vi "HEWH Analyze Total.vi"(7 "Test Type":T6, 8 "error in (no error)":errorcluster, 11 "UEF Calculated Values Input":T1 {"Data Indexes"."15 sec after Draw Index" format="%#.2f"; "Data Indexes"."15 sec after Draw Timestamp" format="%#.2f"; "Data Indexes"."Test Start Timestamp" format="%.2f"; "Data Indexes"."Test End Timestamp" format="%.2f"; "Data Indexes"."T0 Timestamp" format="%.2f"; "Data Indexes"."Tsf Timestamp" format="%.2f"; "Data Indexes"."Tsu0 Timestamp" format="%.2f"; "Data Indexes"."Tmax1 Timestamp" format="%.2f"; "Data Indexes"."Draw Index Timestamp" format="%#.2f"; "Data Indexes"."Non-Draw Timestamp" format="%#.2f"; "Data Indexes"."Heating Timestamp" format="%#.2f"; "Data Indexes"."Start Energy (BTU-Gas)" format="%.6f"; "Data Indexes"."Start Watt Hours" format="%.6f"; "Static Data"."V - Volume of Wh (True)" format="%.5f"; "Static Data"."T-Ambinet Nominal (°F)" format="%.5f"; "Static Data"."T-Inlet Setpoint (°F)" format="%.5f"; "Static Data"."T-Wh Setpoint (°F)" format="%.5f"; "Sampled Data"."Qe (Wh)" format="%.5f"; "Sampled Data"."Tau stby2 (hr)" format="%.5f"; "Sampled Data"."Tastby2 (°F)" format="%.5f"; "Sampled Data"."Qf (BTU)" format="%.5f"; "Sampled Data"."Qe (BTU)" format="%.5f"; "Sampled Data"."Tmax1 (°F)" format="%.5f"; "Sampled Data"."T0 (°F)" format="%.5f"; "Sampled Data"."Qr (BTU)" format="%.5f"; "Sampled Data"."T 24(°F)" format="%.5f"; "Sampled Data"."T astby(°F)" format="%.5f"; "Sampled Data"."T tstby(°F)" format="%.5f"; "Sampled Data"."T su0(°F)" format="%.5f"; "Sampled Data"."T suf(°F)" format="%.5f"; "Sampled Data"."Tau stby_1 (hr)" format="%.5f"; "Sampled Data"."Qsuf (BTU)" format="%.5f"; "Sampled Data"."Qsu0 (BTU)" format="%.5f"; "Calculated Values"."Draw Bonus Volume (gal)" format="%.6f"; "Calculated Values"."Adjustment Factor" format="%.6f"; "Calculated Values"."T*avg_del(n-1)" format="%.6f"; "Calculated Values"."T*min(n-1)" format="%.6f"; "Calculated Values"."T*avg_del(n)" format="%.6f"; "Calculated Values"."Vn" format="%.6f"; "Calculated Values"."Qdm (BTU)" format="%.6f"; "Calculated Values"."QHWD (BTU)" format="%.6f"; "Calculated Values"."QHW (BTU)" format="%.6f"; "Calculated Values"."UEF" format="%.6f"; "Calculated Values"."QHW67 (BTU)" format="%.6f"; "Calculated Values"."Qda (BTU)" format="%.6f"; "Calculated Values"."Qd (BTU)" format="%.6f"; "Calculated Values"."Q (BTU)" format="%.6f"; "Calculated Values"."UA (BTU/(hr*F))" format="%.6f"; "Calculated Values"."Qhr (BTU/hr)" format="%.6f"; "Calculated Values"."Qstby (BTU)" format="%.6f"; "Calculated Values"."nu_r" format="%.6f"; "Calculated Values"."CpUEF (BTU/(lb*F))" format="%.6f"; "Calculated Values"."rho_nu (lb/gal)" format="%.6f"; "Calculated Values"."V1- Vol (Gal)" format="%.6f"; "Calculated Values"."M cluster mass removed (lb)" format="%.6f"; "Calculated Values"."Cp theoretical (BTU/(lbm °F))" format="%.6f"; "Calculated Values"."Tin1 - Mean Inlet 1st Cluster (°F)" format="%.6f"; "Calculated Values"."Tdel1-Mean Outlet 1st Cluster(°F)" format="%.6f"; "Calculated Values"."Cp 24 (BTU/(lb*F))" format="%.6f"; "Calculated Values"."Cp standby (BTU/(lb*F))" format="%.6f"; "Calculated Values"."Cp2 (BTU/(lb*F))" format="%.6f"; "Calculated Values"."Cp1 (BTU/(lb*F))" format="%.6f"; "Calculated Values"."rho 24 (lb/gal)" format="%.6f"; "Calculated Values"."rho standby (lb/gal)" format="%.6f"; "Calculated Values"."rho 2 (lb/gal)" format="%.6f"; "Calculated Values"."Density of cold water All (lbm/gal)" format="%#.3g"; "Calculated Values"."CpHW (BTU/(lbm °F))" format="%#.3g"; "Calculated Values"."Density of hot water All (lbm/gal)" format="%#.3g"; "Calculated Values"."Mass of water All (lbm)" format="%#.3f"}) -> (0 "error out":errorcluster, 3 "UEF Calculated Values Output":T1 {"Data Indexes"."15 sec after Draw Index" format="%#.2f"; "Data Indexes"."15 sec after Draw Timestamp" format="%#.2f"; "Data Indexes"."Test Start Timestamp" format="%.2f"; "Data Indexes"."Test End Timestamp" format="%.2f"; "Data Indexes"."T0 Timestamp" format="%.2f"; "Data Indexes"."Tsf Timestamp" format="%.2f"; "Data Indexes"."Tsu0 Timestamp" format="%.2f"; "Data Indexes"."Tmax1 Timestamp" format="%.2f"; "Data Indexes"."Draw Index Timestamp" format="%#.2f"; "Data Indexes"."Non-Draw Timestamp" format="%#.2f"; "Data Indexes"."Heating Timestamp" format="%#.2f"; "Data Indexes"."Start Energy (BTU-Gas)" format="%.6f"; "Data Indexes"."Start Watt Hours" format="%.6f"; "Static Data"."V - Volume of Wh (True)" format="%.5f"; "Static Data"."T-Ambinet Nominal (°F)" format="%.5f"; "Static Data"."T-Inlet Setpoint (°F)" format="%.5f"; "Static Data"."T-Wh Setpoint (°F)" format="%.5f"; "Sampled Data"."Qe (Wh)" format="%.5f"; "Sampled Data"."Tau stby2 (hr)" format="%.5f"; "Sampled Data"."Tastby2 (°F)" format="%.5f"; "Sampled Data"."Qf (BTU)" format="%.5f"; "Sampled Data"."Qe (BTU)" format="%.5f"; "Sampled Data"."Tmax1 (°F)" format="%.5f"; "Sampled Data"."T0 (°F)" format="%.5f"; "Sampled Data"."Qr (BTU)" format="%.5f"; "Sampled Data"."T 24(°F)" format="%.5f"; "Sampled Data"."T astby(°F)" format="%.5f"; "Sampled Data"."T tstby(°F)" format="%.5f"; "Sampled Data"."T su0(°F)" format="%.5f"; "Sampled Data"."T suf(°F)" format="%.5f"; "Sampled Data"."Tau stby_1 (hr)" format="%.5f"; "Sampled Data"."Qsuf (BTU)" format="%.5f"; "Sampled Data"."Qsu0 (BTU)" format="%.5f"; "Calculated Values"."Draw Bonus Volume (gal)" format="%.6f"; "Calculated Values"."Adjustment Factor" format="%.6f"; "Calculated Values"."T*avg_del(n-1)" format="%.6f"; "Calculated Values"."T*min(n-1)" format="%.6f"; "Calculated Values"."T*avg_del(n)" format="%.6f"; "Calculated Values"."Vn" format="%.6f"; "Calculated Values"."Qdm (BTU)" format="%.6f"; "Calculated Values"."QHWD (BTU)" format="%.6f"; "Calculated Values"."QHW (BTU)" format="%.6f"; "Calculated Values"."UEF" format="%.6f"; "Calculated Values"."QHW67 (BTU)" format="%.6f"; "Calculated Values"."Qda (BTU)" format="%.6f"; "Calculated Values"."Qd (BTU)" format="%.6f"; "Calculated Values"."Q (BTU)" format="%.6f"; "Calculated Values"."UA (BTU/(hr*F))" format="%.6f"; "Calculated Values"."Qhr (BTU/hr)" format="%.6f"; "Calculated Values"."Qstby (BTU)" format="%.6f"; "Calculated Values"."nu_r" format="%.6f"; "Calculated Values"."CpUEF (BTU/(lb*F))" format="%.6f"; "Calculated Values"."rho_nu (lb/gal)" format="%.6f"; "Calculated Values"."V1- Vol (Gal)" format="%.6f"; "Calculated Values"."M cluster mass removed (lb)" format="%.6f"; "Calculated Values"."Cp theoretical (BTU/(lbm °F))" format="%.6f"; "Calculated Values"."Tin1 - Mean Inlet 1st Cluster (°F)" format="%.6f"; "Calculated Values"."Tdel1-Mean Outlet 1st Cluster(°F)" format="%.6f"; "Calculated Values"."Cp 24 (BTU/(lb*F))" format="%.6f"; "Calculated Values"."Cp standby (BTU/(lb*F))" format="%.6f"; "Calculated Values"."Cp2 (BTU/(lb*F))" format="%.6f"; "Calculated Values"."Cp1 (BTU/(lb*F))" format="%.6f"; "Calculated Values"."rho 24 (lb/gal)" format="%.6f"; "Calculated Values"."rho standby (lb/gal)" format="%.6f"; "Calculated Values"."rho 2 (lb/gal)" format="%.6f"; "Calculated Values"."Density of cold water All (lbm/gal)" format="%#.3g"; "Calculated Values"."CpHW (BTU/(lbm °F))" format="%#.3g"; "Calculated Values"."Density of hot water All (lbm/gal)" format="%#.3g"; "Calculated Values"."Mass of water All (lbm)" format="%#.3f"})   [LabVIEW 2023]
uses:
  Type Definitions/UEF Constants.ctl
  Type Definitions/HEWH Draw Stats.ctl
  Type Definitions/HEWH FHR Draw Type.ctl
  Type Definitions/FHR Bins.ctl
  Type Definitions/HEWH Meter Type.ctl
  Type Definitions/HEWH Test Type.ctl
  <vilib>/Utility/error.llb/whitespace.ctl
  <vilib>/Utility/error.llb/Trim Whitespace One-Sided.vi
panel:
  out "Sampled Data.Hot Water Draw Amounts-(Gal)":dbl[](array[numeric])
  out "output variable":dbl
  # "FHR"
  # "FHR"
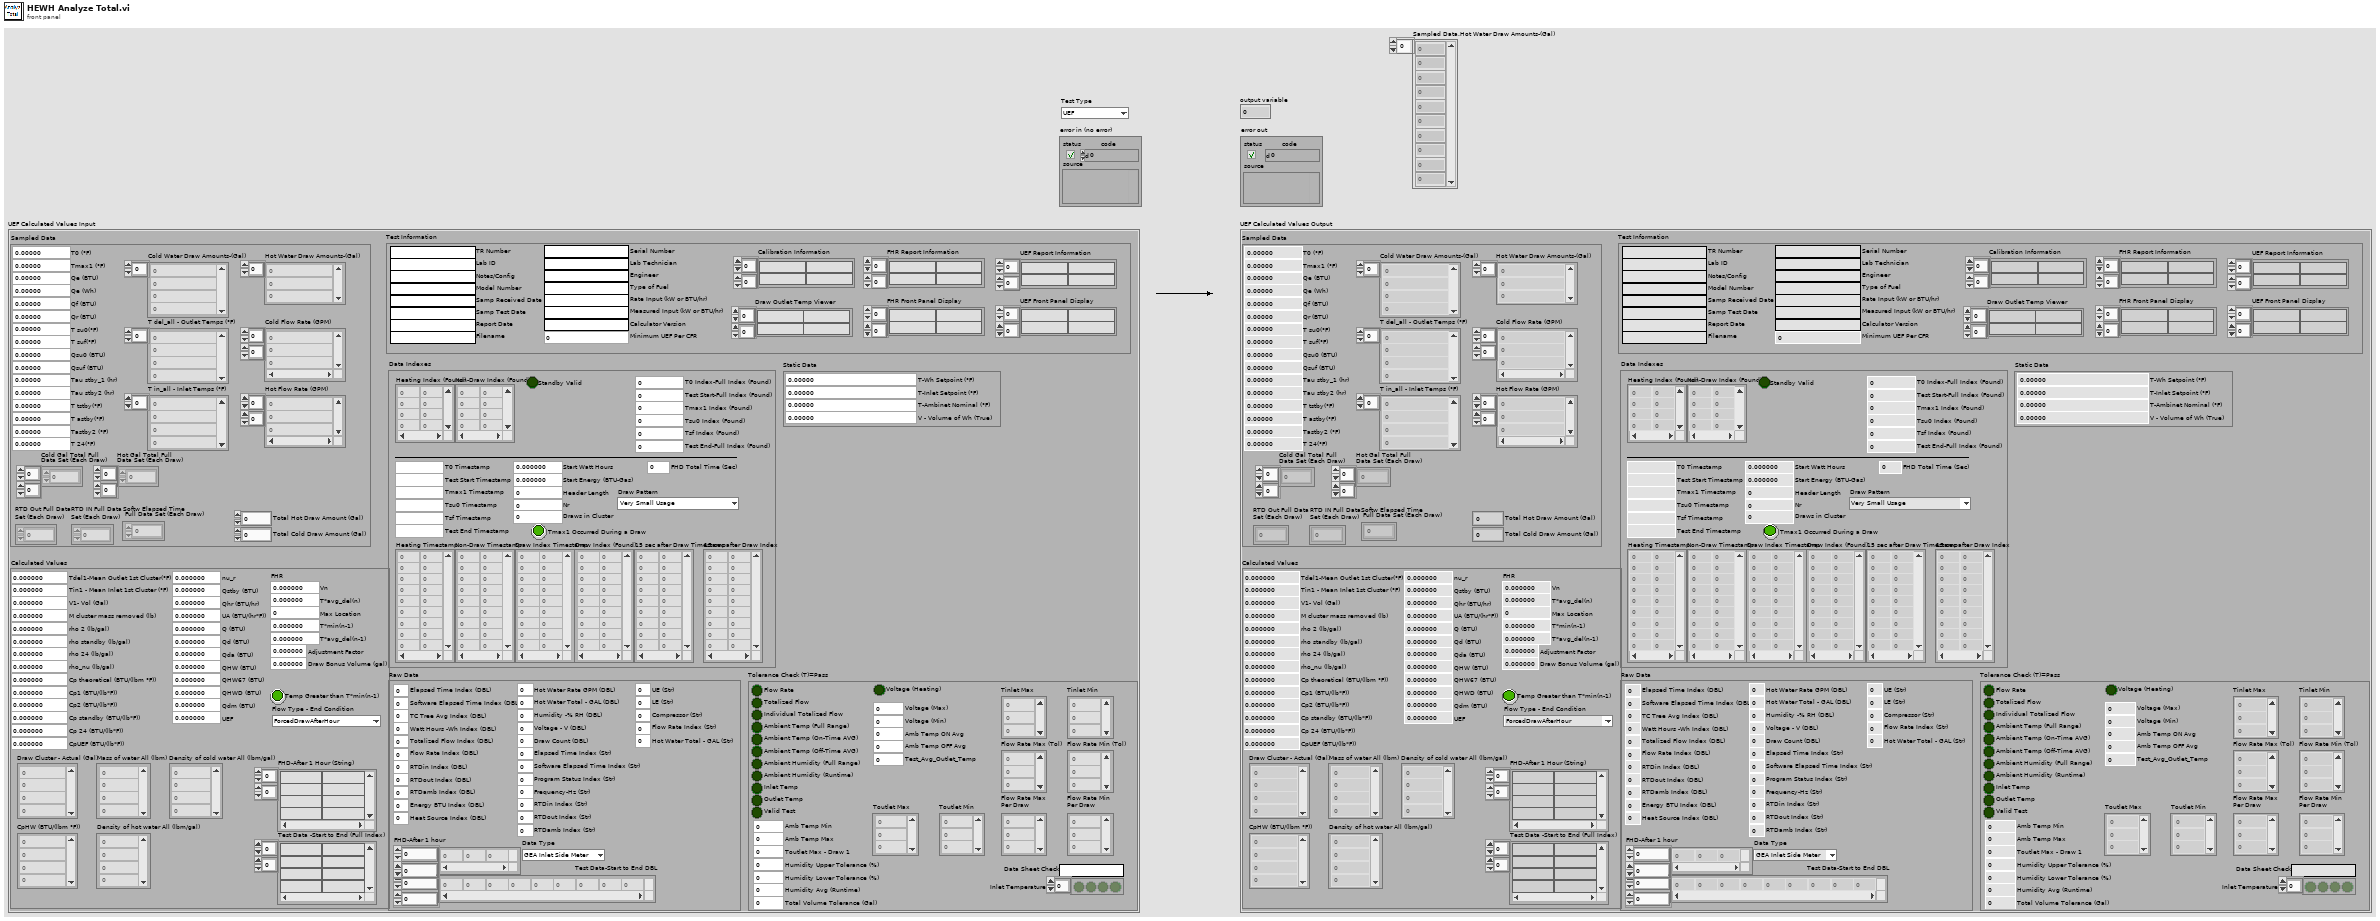
[diagram p1: front panel]
types:
  T1 = typedef "UEF Constants.ctl" = cluster{"Calculated Values":T2, "Sampled Data":cluster{"Cold Water Draw Amounts-(Gal)":dbl[], "T del_all - Outlet Temps (°F)":dbl[], "T in_all - Inlet Temps (°F)":dbl[], "Qsu0 (BTU)":dbl, "Qsuf (BTU)":dbl, "Tau stby_1 (hr)":dbl, "T suf(°F)":dbl, "T su0(°F)":dbl, "T tstby(°F)":dbl, "T astby(°F)":dbl, "T 24(°F)":dbl, "Qr (BTU)":dbl, "T0 (°F)":dbl, "Tmax1 (°F)":dbl, "Qe (BTU)":dbl, "Qf (BTU)":dbl, "Tastby2 (°F)":dbl, "RTD Out Full Data\nSet (Each Draw)":dbl[][], "RTD IN Full Data\nSet (Each Draw)":dbl[][], "Tau stby2 (hr)":dbl, "Hot Water Draw Amounts-(Gal)":dbl[], "Cold Flow Rate (GPM)":dbl[][], "Hot Flow Rate (GPM)":dbl[][], "Softw Elapsed Time\n Full Data Set (Each Draw)":dbl[][], "Cold Gal Total Full\nData Set (Each Draw)":dbl[][], "Total Hot Draw Amount (Gal) ":dbl, "Total Cold Draw Amount (Gal)":dbl, "Qe (Wh)":dbl, "Hot Gal Total Full\nData Set (Each Draw)":dbl[][]}, "Static Data":cluster{"T-Wh Setpoint (°F)":dbl, "T-Inlet Setpoint (°F)":dbl, "T-Ambinet Nominal (°F)":dbl, "V - Volume of Wh (True)":dbl}, "Data Indexes":cluster{"Test Start-Full Index (Found)":i32, "Header Length":i32, "Draw Index (Found)":i32[][], "Nr":i32, "Start Watt Hours":dbl, "Tsu0 Index (Found)":i32, "Tsf Index (Found)":i32, "Start Energy (BTU-Gas)":dbl, "Draws in Cluster":i32, "T0 Index-Full Index (Found)":i32, "Non-Draw Index (Found)":i32[][], "Tmax1 Index (Found)":i32, "Test End-Full Index (Found)":i32, "Heating Index (Found)":i32[][], "Heating Timestamp":dbl[][], "Non-Draw Timestamp":dbl[][], "Draw Index Timestamp":dbl[][], "Tmax1 Timestamp":dbl, "Tsu0 Timestamp":dbl, "Tsf Timestamp":dbl, "T0 Timestamp":dbl, "Test End Timestamp":dbl, "Test Start Timestamp":dbl, "15 sec after Draw Timestamp":dbl[][], "15 sec after Draw Index":dbl[][], "Tmax1 Occurred During a Draw":bool, "FHD Total Time (Sec)":dbl, "Draw Pattern":T4, "Standby Valid":bool}, "Raw Data":cluster{"Elapsed Time Index (DBL)":i32, "Software Elapsed Time Index (DBL)":i32, "TC Tree Avg Index (DBL)":i32, "Watt Hours -Wh Index (DBL)":i32, "Energy BTU Index (DBL)":i32, "Totalized Flow Index (DBL)":i32, "Flow Rate Index (DBL)":i32, "Program Status Index (Str)":i32, "RTDin Index (DBL)":i32, "RTDout Index (DBL)":i32, "RTDamb Index (DBL)":i32, "Test Data-Start to End DBL":dbl[][], "Data Type":T5, "Heat Source Index (DBL)":i32, "Hot Water Rate GPM (DBL)":i32, "Hot Water Total - GAL (DBL)":i32, "FHD-After 1 hour":dbl[][], "Humidity -% RH (DBL)":i32, "Voltage - V (DBL)":i32, "Draw Count (DBL)":i32, "Elapsed Time Index (Str)":i32, "Software Elapsed Time Index (Str)":i32, "Frequency-Hz (Str)":i32, "RTDin Index (Str)":i32, "RTDout Index (Str)":i32, "RTDamb Index (Str)":i32, "UE (Str)":i32, "LE (Str)":i32, "Compressor (Str)":i32, "Flow Rate Index (Str)":i32, "Hot Water Total - GAL (Str)":i32}, "Tolerance Check (T)=Pass":cluster{"Flow Rate":bool, "Totalized Flow":bool, "Ambient Temp (Full Range)":bool, "Ambient Humidity (Full Range)":bool, "Inlet Temp":bool, "Outlet Temp":bool, "Valid Test":bool, "Individual Totalized Flow":bool, "Data Sheet Check":string, "Inlet Temperature":bool[], "Tinlet Max":dbl[], "Tinlet Min":dbl[], "Flow Rate Max (Tol)":dbl[], "Flow Rate Min (Tol)":dbl[], "Amb Temp Max":dbl, "Amb Temp Min":dbl, "Toutlet Max - Draw 1":dbl, "Humidity Upper Tolerance (%)":dbl, "Total Volume Tolerance (Gal)":dbl, "Humidity Lower Tolerance (%)":dbl, "Flow Rate Max\nPer Draw":dbl[], "Flow Rate Min\nPer Draw":dbl[], "Ambient Humidity (Runtime)":bool, "Humidity Avg (Runtime)":dbl, "Ambient Temp (On-Time AVG)":bool, "Ambient Temp (Off-Time AVG)":bool, "Amb Temp OFF Avg":dbl, "Amb Temp ON Avg":dbl, "Voltage (Heating)":bool, "Voltage (Min)":dbl, "Voltage (Max)":dbl, "Toutlet Max":dbl[], "Toutlet Min":dbl[], "Test_Avg_Outlet_Temp":dbl}, "Test Information":cluster{"TR Number":string, "Lab ID":string, "Notes/Config":string, "Model Number":string, "Serial Number":string, "Lab Technician":string, "Engineer":string, "Type of Fuel":string, "Samp Received Date":string, "Samp Test Date":string, "Report Date":string, "Rate Input (kW or BTU/hr)":string, "Measured Input (kW or BTU/hr)":string, "Filename":string, "Calibration Information":string[][], "Calculator Version":string, "Minimum UEF Per CFR":dbl, "UEF Report Information":string[][], "FHR Report Information":string[][], "FHR Front Panel Display":string[][], "UEF Front Panel Display":string[][], "Draw Outlet Temp Viewer":string[][]}}
  T2 = typedef "HEWH Draw Stats.ctl" = cluster{"Draw Cluster - Actual (Gal)":dbl[], "Mass of water All (lbm)":dbl[], "Density of hot water All (lbm/gal)":dbl[], "CpHW (BTU/(lbm °F))":dbl[], "rho 2 (lb/gal)":dbl, "rho standby (lb/gal)":dbl, "rho 24 (lb/gal)":dbl, "Cp1 (BTU/(lb*F))":dbl, "Cp2 (BTU/(lb*F))":dbl, "Cp standby (BTU/(lb*F))":dbl, "Cp 24 (BTU/(lb*F))":dbl, "nu_r":dbl, "Qstby (BTU)":dbl, "Qhr (BTU/hr)":dbl, "UA (BTU/(hr*F))":dbl, "Q (BTU)":dbl, "Qd (BTU)":dbl, "Qda (BTU)":dbl, "QHW67 (BTU)":dbl, "UEF":dbl, "Tdel1-Mean Outlet 1st Cluster(°F)":dbl, "Tin1 - Mean Inlet 1st Cluster (°F)":dbl, "Cp theoretical (BTU/(lbm °F))":dbl, "M cluster mass removed (lb)":dbl, "V1- Vol (Gal)":dbl, "Test Data -Start to End (Full Index)":string[][], "rho_nu (lb/gal)":dbl, "Density of cold water All (lbm/gal)":dbl[], "CpUEF (BTU/(lb*F))":dbl, "QHW (BTU)":dbl, "QHWD (BTU)":dbl, "Qdm (BTU)":dbl, "FHD-After 1 Hour (String)":string[][], "Vn":dbl, "T*avg_del(n)":dbl, "Max Location":i32, "T*min(n-1)":dbl, "T*avg_del(n-1)":dbl, "Temp Greater than T*min(n-1)":bool, "Adjustment Factor":dbl, "Draw Bonus Volume (gal)":dbl, "Flow Type - End Condition":T3}
  T3 = typedef "HEWH FHR Draw Type.ctl" = enum16{"ForcedDrawAfterHour", "HeatingCutoffBeforeHour"}
  T4 = typedef "FHR Bins.ctl" = enum16{"Very Small Usage", "Low Usage", "Medium Usage", "High Usage", "Undefined"}
  T5 = typedef "HEWH Meter Type.ctl" = enum16{"GEA Inlet Side Meter", "GEA Outlet Side Meter", "CSA Inlet Side Meter"}
  T6 = typedef "HEWH Test Type.ctl" = enum16{"UEF", "FHD"}
  T7 = typedef "whitespace.ctl" = u16
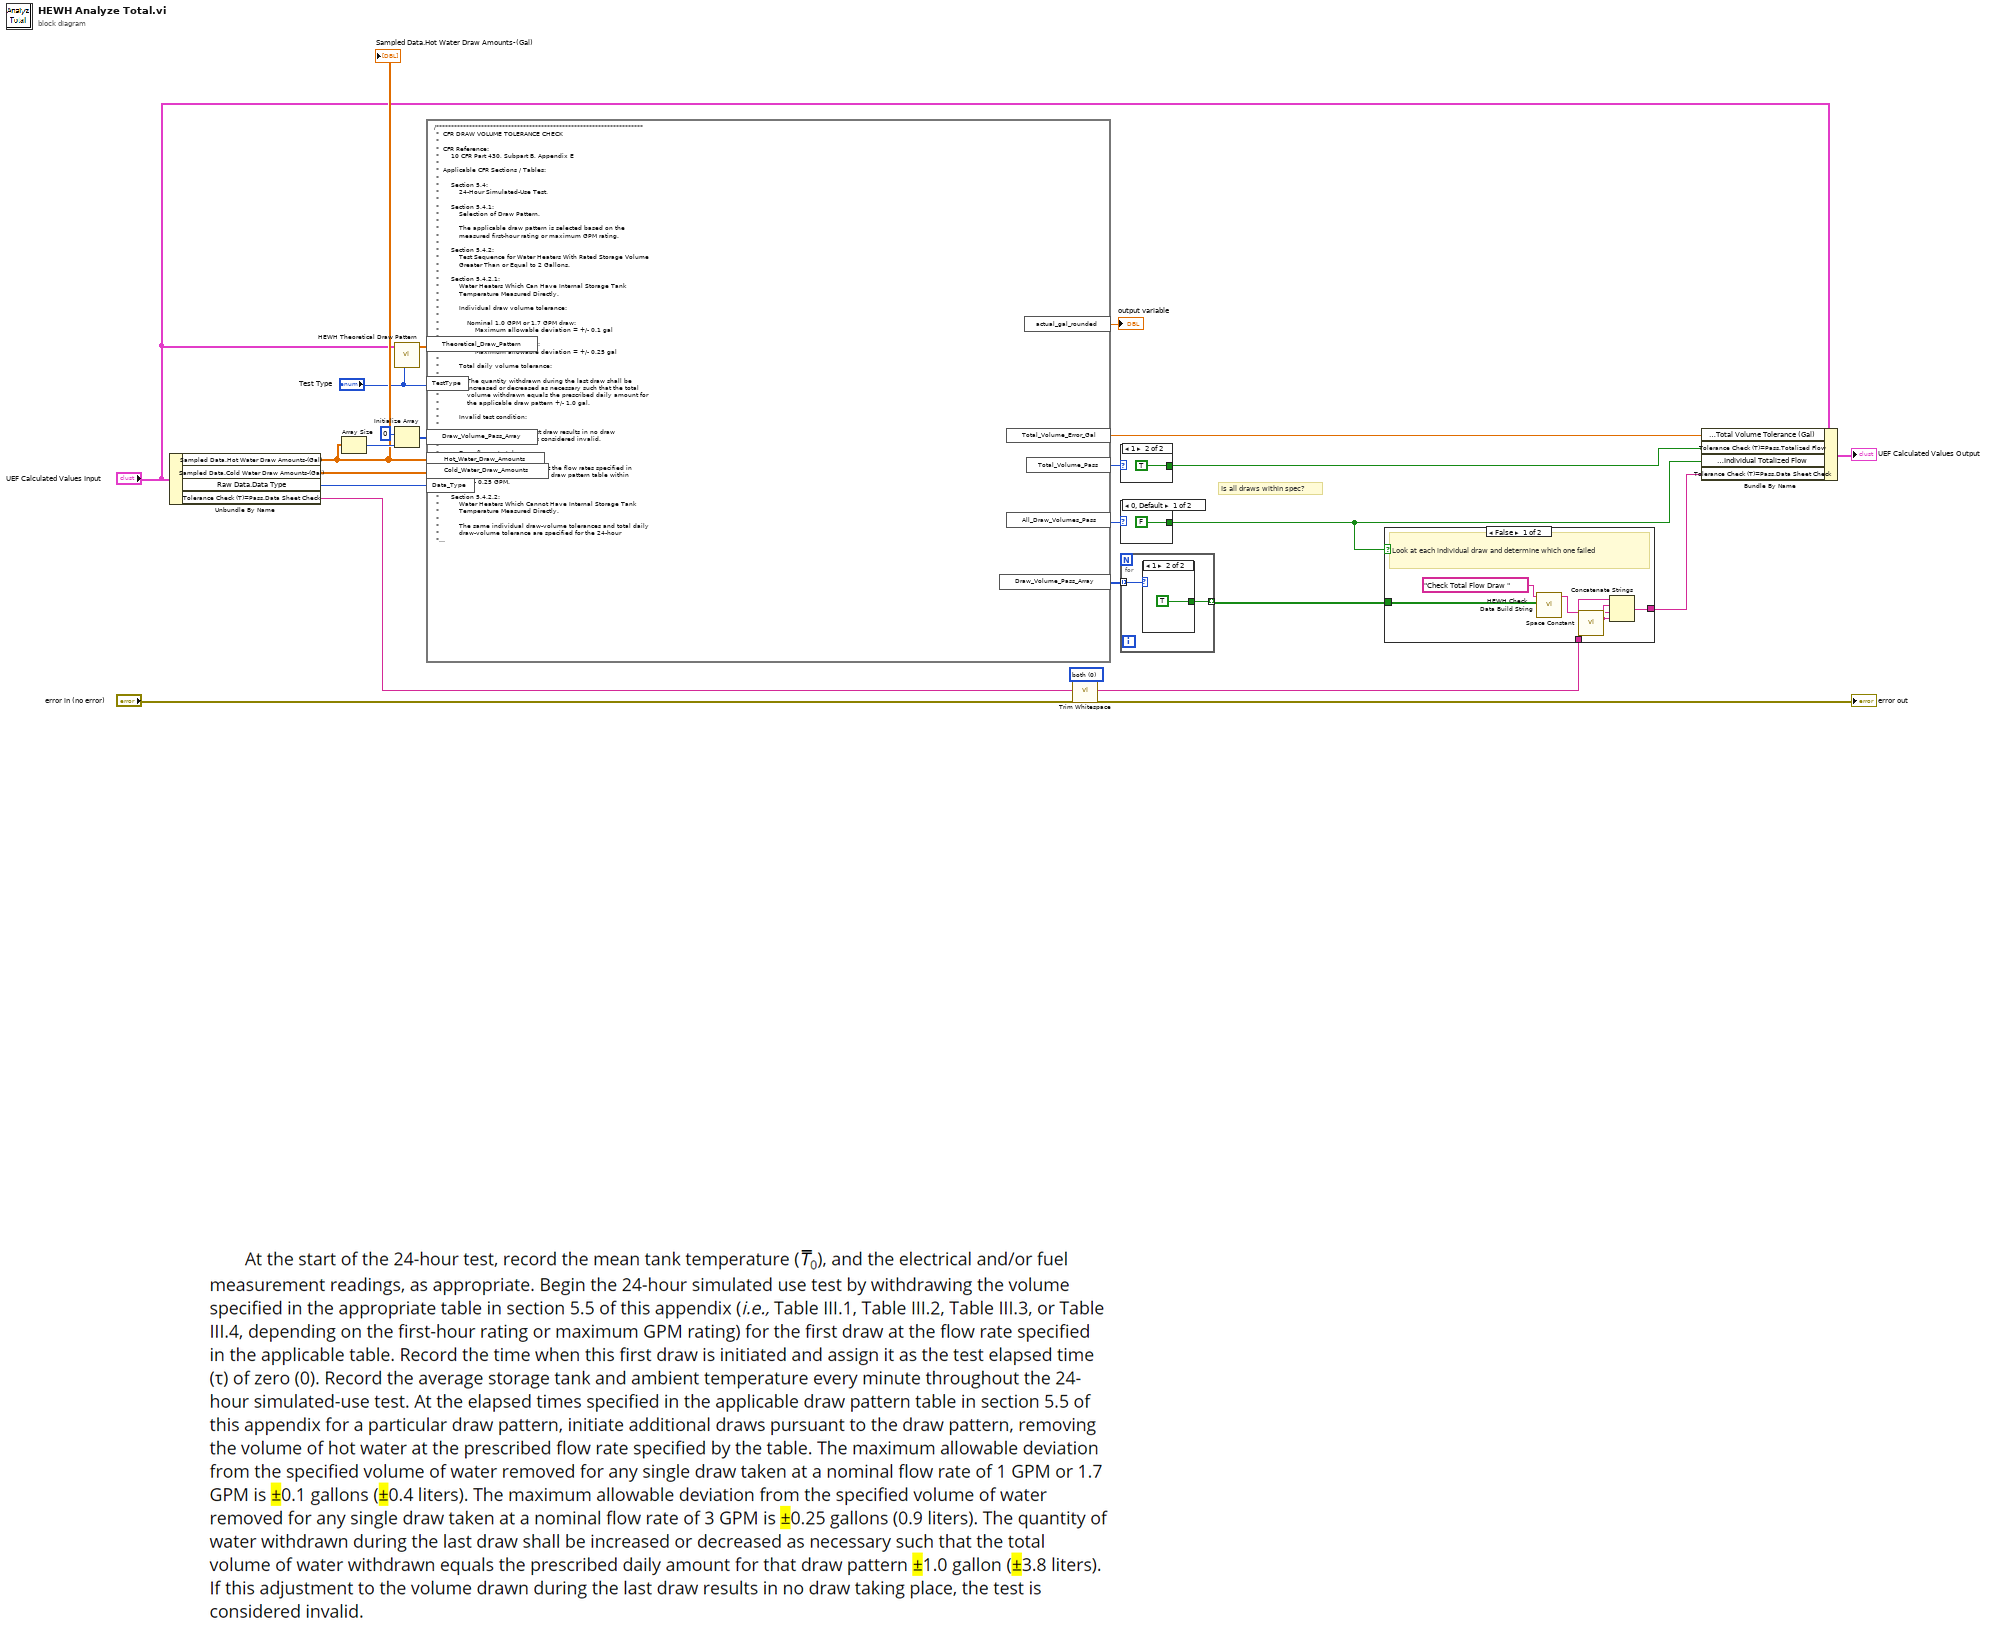
[diagram p0: block diagram]
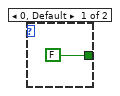
[diagram p3: hidden frame]
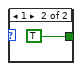
[diagram p4: hidden frame]
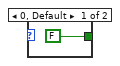
[diagram p5: hidden frame]
diagram:
  w10 = T7 0 items=["both", "start of string", "end of string"] ("location (both)")
  # "Is all draws within spec?"
  n1 = Unbundle By Name("UEF Calculated Values Input") -> ("Sampled Data.Hot Water Draw Amounts-(Gal)"=w14:dbl[], "Sampled Data.Cold Water Draw Amounts-(Gal)"=w2:dbl[], "Raw Data.Data Type"=w3:T5, "Tolerance Check (T)=Pass.Data Sheet Check"=w9:string)
  "Sampled Data.Hot Water Draw Amounts-(Gal)" <- w14
  n2 = Array Size(array=w14) -> (size(s)=w21:i32)
  n3 = call "HEWH Theoretical Draw Pattern.vi"("Test Type"="Test Type", "UEF Calculated Values Input"="UEF Calculated Values Input") -> ("Theoretical Draw Pattern"=w13:dbl[][])  [unwired: 8 in, 1 out]
  n4 = Initialize Array(u8 0, w21) -> (w20:u8[])
  n5 = formula code="/*********************************************************************\n *  CFR DRAW VOLUME TOLERANCE CHECK\n *\n *  CFR Reference:\n *      10 CFR Part 430, Subpart B, Appendix E\n *\n *  Applicable CFR Sections / Tables:\n *\n *      Section 5.4:\n *          24-Hour Simulated-Use Test.\n *\n *      Section 5.4.1:\n *          Selection of Draw Pattern.\n *\n *          The applicable draw pattern is selected based on the\n *          measured first-hour rating or maximum GPM rating.\n *\n *      Section 5.4.2:\n *          Test Sequence for Water Heaters With Rated Storage Volume\n *          Greater Than or Equal to 2 Gallons.\n *\n *      Section 5.4.2.1:\n *          Water Heaters Which Can Have Internal Storage Tank\n *          Temperature Measured Directly.\n *\n *          Individual draw volume tolerance:\n *\n *              Nominal 1.0 GPM or 1.7 GPM draw:\n *                  Maximum allowable deviation = +/- 0.1 gal\n *\n *              Nominal 3.0 GPM draw:\n *                  Maximum allowable deviation = +/- 0.25 gal\n *\n *          Total daily volume tolerance:\n *\n *              The quantity withdrawn during the last draw shall be\n *              increased or decreased as necessary such that the total\n *              volume withdrawn equals the prescribed daily amount for\n *              the applicable draw pattern +/- 1.0 gal.\n *\n *          Invalid test condition:\n *\n *              If adjustment of the last draw results in no draw\n *              taking place, the test is considered invalid.\n *\n *          Draw flow-rate tolerance:\n *\n *              All draws shall be made at the flow rates specified in\n *              the applicable Section 5.5 draw pattern table within\n *              +/- 0.25 GPM.\n *\n *      Section 5.4.2.2:\n *          Water Heaters Which Cannot Have Internal Storage Tank\n *          Temperature Measured Directly.\n *\n *          The same individual draw-volume tolerances and total daily\n *          draw-volume tolerance are specified for the 24-hour\n *          simulated-use test.\n *\n *      Section 5.5:\n *          Draw Patterns.\n *\n *      Table III.1:\n *          Very-Small-Usage Draw Pattern\n *\n *      Table III.2:\n *          Low-Usage Draw Pattern\n *\n *      Table III.3:\n *          Medium-Usage Draw Pattern\n *\n *      Table III.4:\n *          High-Usage Draw Pattern\n *\n *  Inputs:\n *      Hot_Water_Draw_Amounts[]       // Actual measured hot-water draw volumes, gal\n *      Cold_Water_Draw_Amounts[]      // Actual measured cold-water draw volumes, gal\n *      Theoretical_Draw_Pattern[][]   // Column 0 = prescribed draw volume, gal\n *                                     // Column 1 = prescribed flow rate, GPM\n *\n *      TestType                       // 0 = run CFR draw-volume check\n *                                     // 1 = bypass check and force pass\n *\n *      Data_Type                      // 0 = use Hot_Water_Draw_Amounts\n *                                     // 1 = use Cold_Water_Draw_Amounts\n *\n *  Outputs:\n *      Total_Volume_Error_Gal         // Signed difference:\n *                                     // Total_Actual - Theoretical_Total, gal\n *\n *      Total_Volume_Pass              // 1 = total volume within +/- 1.0 gal\n *\n *      All_Draw_Volumes_Pass          // 1 = all individual draws pass\n *\n *      Draw_Volume_Pass_Array[]       // Per-draw pass/fail array:\n *                                     // 1 = pass, 0 = fail\n *\n *  Assumption:\n *      Theoretical_Draw_Pattern uses only CFR Section 5.5\n *      draw-pattern flow rates applicable to this check:\n *          1.0 GPM, 1.7 GPM, and 3.0 GPM.\n *********************************************************************/\n\n\n/* -------------------- Local Variables -------------------- */\n\nint32 i;\nint32 N;\n\nfloat theoretical_gal;\nfloat actual_gal;\nfloat theoretical_flow;\nfloat draw_tol;\nfloat draw_error;\n\nfloat Theoretical_Total;\nfloat Total_Actual;\nfloat Lower_Limit_Total;\nfloat Upper_Limit_Total;\nfloat actual_gal_rounded;\n\n\n/* -------------------- Defaults -------------------- */\n\nTheoretical_Total = 0.0;\nTotal_Actual = 0.0;\n\nLower_Limit_Total = 0.0;\nUpper_Limit_Total = 0.0;\n\nTotal_Volume_Error_Gal = 0.0;\n\nint32 Total_Volume_Pass = 0;\nint32 All_Draw_Volumes_Pass = 1;\n\n\n/* -------------------- Determine Array Length --------------------\n *\n * Data_Type basis:\n *\n *      Data_Type = 0:\n *          Use Hot_Water_Draw_Amounts.\n *\n *      Data_Type = 1:\n *          Use Cold_Water_Draw_Amounts.\n */\n\nif (Data_Type == 0)\n{\n    N = sizeOfDim(Hot_Water_Draw_Amounts, 0);\n}\nelse\n{\n    N = sizeOfDim(Cold_Water_Draw_Amounts, 0);\n}\n\n\n/* -------------------- Test Type Bypass Check --------------------\n *\n * TestType basis:\n *\n *      TestType = 0:\n *          Run the normal CFR draw-volume tolerance check.\n *\n *      TestType = 1:\n *          Bypass the CFR draw-volume tolerance check.\n *          Force total volume, all individual draw volumes, and each\n *          element of Draw_Volume_Pass_Array to pass.\n */\n\nif (TestType == 0)\n{\n\n    /* -------------------- Sum Actual and Prescribed Volumes -------------------- */\n\n    for (i = 0; i < N; i++)\n    {\n        /*\n         * Select the actual measured draw volume based on Data_Type.\n         *\n         *      Data_Type = 0:\n         *          Use hot-water draw volume.\n         *\n         *      Data_Type = 1:\n         *          Use cold-water draw volume.\n         */\n\n        if (Data_Type == 0)\n        {\n            actual_gal = Hot_Water_Draw_Amounts[i];\n        }\n        else\n        {\n            actual_gal = Cold_Water_Draw_Amounts[i];\n        }\n\n        theoretical_gal = Theoretical_Draw_Pattern[i][0];\n\n        Total_Actual += actual_gal;\n        Theoretical_Total += theoretical_gal;\n    }\n\n\n    /* -------------------- Total Daily Volume Check --------------------\n     *\n     * CFR basis:\n     *      10 CFR Part 430, Subpart B, Appendix E,\n     *      Section 5.4.2.1\n     *\n     *      The quantity withdrawn during the last draw shall be\n     *      increased or decreased as necessary such that the total\n     *      volume withdrawn equals the prescribed daily amount for the\n     *      applicable draw pattern +/- 1.0 gallon.\n     *\n     *      If adjustment of the last draw results in no draw taking\n     *      place, the test is considered invalid.\n     *\n     * Note:\n     *      This code checks the final total-volume tolerance only.\n     *      It does not independently determine whether adjustment of\n     *      the last draw resulted in no draw taking place.\n     */\n\n    Lower_Limit_Total = Theoretical_Total - 1.0;\n    Upper_Limit_Total = Theoretical_Total + 1.0;\n\n    Total_Volume_Error_Gal = Total_Actual - Theoretical_Total;\n\n    if (Total_Actual >= Lower_Limit_Total && Total_Actual <= Upper_Limit_Total)\n    {\n        Total_Volume_Pass = 1;\n    }\n    else\n    {\n        Total_Volume_Pass = 0;\n    }\n\n\n    /* -------------------- Individual Draw Volume Checks --------------------\n     *\n     * CFR basis:\n     *      10 CFR Part 430, Subpart B, Appendix E,\n     *      Section 5.4.2.1\n     *\n     *      For any single draw taken at a nominal flow rate of\n     *      1.0 GPM or 1.7 GPM:\n     *\n     *          Maximum allowable deviation = +/- 0.1 gal\n     *\n     *      For any single draw taken at a nominal flow rate of\n     *      3.0 GPM:\n     *\n     *          Maximum allowable deviation = +/- 0.25 gal\n     */\n\n    for (i = 0; i < N; i++)\n    {\n        theoretical_gal = Theoretical_Draw_Pattern[i][0];\n        theoretical_flow = Theoretical_Draw_Pattern[i][1];\n\n        /*\n         * Select the actual measured draw volume based on Data_Type.\n         *\n         *      Data_Type = 0:\n         *          Use hot-water draw volume.\n         *\n         *      Data_Type = 1:\n         *          Use cold-water draw volume.\n         */\n\n        if (Data_Type == 0)\n        {\n            actual_gal = Hot_Water_Draw_Amounts[i];\n        }\n        else\n        {\n            actual_gal = Cold_Water_Draw_Amounts[i];\n        }\n        /*\n         * Round the measured individual draw volume to two decimal\n         * places before applying the individual draw-volume tolerance.\n         */\n        actual_gal_rounded = floor(actual_gal * 100.0 + 0.5) / 100.0;\n\n        if (theoretical_flow == 1.0 || theoretical_flow == 1.7)\n        {\n            draw_tol = 0.1;\n        }\n        else if (theoretical_flow == 3.0)\n        {\n            draw_tol = 0.25;\n        }\n        else\n        {\n            /*\n             * This condition should not occur when\n             * Theoretical_Draw_Pattern contains only the prescribed\n             * CFR Section 5.5 flow rates applicable to this check.\n             */\n            draw_tol = 0.0;\n        }\n\n        draw_error = abs(actual_gal_rounded - theoretical_gal);\n\n        if (draw_error <= draw_tol)\n        {\n            Draw_Volume_Pass_Array[i] = 1;\n        }\n        else\n        {\n            Draw_Volume_Pass_Array[i] = 0;\n            All_Draw_Volumes_Pass = 0;\n        }\n    }\n}\nelse\n{\n    /*\n     * TestType = 1:\n     *\n     *      Bypass the CFR draw-volume tolerance check.\n     *      Force all draw-volume outputs to pass.\n     */\n\n    Total_Volume_Pass = 1;\n    All_Draw_Volumes_Pass = 1;\n    Total_Volume_Error_Gal = 0.0;\n\n    for (i = 0; i < N; i++)\n    {\n        Draw_Volume_Pass_Array[i] = 1;\n    }\n}"("Hot_Water_Draw_Amounts"=w14, "Theoretical_Draw_Pattern"=w13, "Draw_Volume_Pass_Array"=w20, "TestType"="Test Type", "Data_Type"=w3, "Cold_Water_Draw_Amounts"=w2) -> ("Total_Volume_Error_Gal"=w15:dbl, "Total_Volume_Pass"=w19:i32, "All_Draw_Volumes_Pass"=w18:i32, "Draw_Volume_Pass_Array"=w17:u8[], "actual_gal_rounded"=→"output variable":dbl)
  n6 = call <vilib>:"Trim Whitespace.vi"("string"=w9, "location (both)"=w10) -> ("trimmed string"=w8:string)
  n7 = case shown="1" w19 {
    tunnel: [FALSE TRUE] -> w16
    frame 0, Default {
    }
    frame 1 {
    }
  }
  n8 = case shown="0, Default" w18 {
    tunnel: [FALSE TRUE] -> w4
    frame 0, Default {
    }
    frame 1 {
    }
  }
  n9 = for {
    tunnel: w17 -> [w29] mode=indexing
    tunnel: [w28] -> w6 mode=indexing
    n10 = case shown="1" w29 {
      tunnel: [FALSE TRUE] -> w28
      frame 0, Default {
      }
      frame 1 {
      }
    }
  }
  n11 = case shown="False" w4 {
    tunnel: w8 -> [w35 w38]
    tunnel: [w33 w38] -> w7
    tunnel: w6 -> [w32 _]
    frame False {
      # "Look at each individual draw and determine which one failed"
      n12 = call "HEWH Check Data Build String.vi"("Check Array"=w32, "Error Input"="Check Total Flow Draw ") -> ("Error Output"=w34:string)  [unwired: 8 in, 1 out]
      n13 = call <vilib>:"Space Constant.vi"() -> ("String"=w36:string)
      n14 = Concatenate Strings(w35, w36, w34, w36) -> (w33:string)
    }
    frame True {
    }
  }
  n15 = Bundle By Name(cluster="UEF Calculated Values Input", "Tolerance Check (T)=Pass.Total Volume Tolerance (Gal)"=w15, "Tolerance Check (T)=Pass.Totalized Flow"=w16, "Tolerance Check (T)=Pass.Individual Totalized Flow"=w4, "Tolerance Check (T)=Pass.Data Sheet Check"=w7) -> (→"UEF Calculated Values Output":T1)
  "error out" <- "error in (no error)"
